vi "Read Attributes.vi"(0 "Linked List in":refnum<class "Linked List.lvclass">, 1 "Linked List ID":string, 3 "Include Private?":bool, 5 "Attribute Names":string[](array[string]), 9 "Flatten Pointer?":bool, 11 "error in (no error)":errorcluster) -> (4 "Linked List out":refnum<class "Linked List.lvclass">, 6 "Attribute Names out":string[](array[string]), 8 "Missing GUIDs out":string[](array[string]), 10 "Attributes":variant[](array[variant]), 12 "Found?":bool[](array[boolean]), 14 "Data IDs":string[](array[string]), 15 "error out":errorcluster)   [LabVIEW 2020, in "Linked Lists.lvlib" / "Linked List.lvclass"]
uses:
  <vilib>/gpm_packages/@cs/linked-list/Source/Linked List/Linked List/Linked List.lvclass
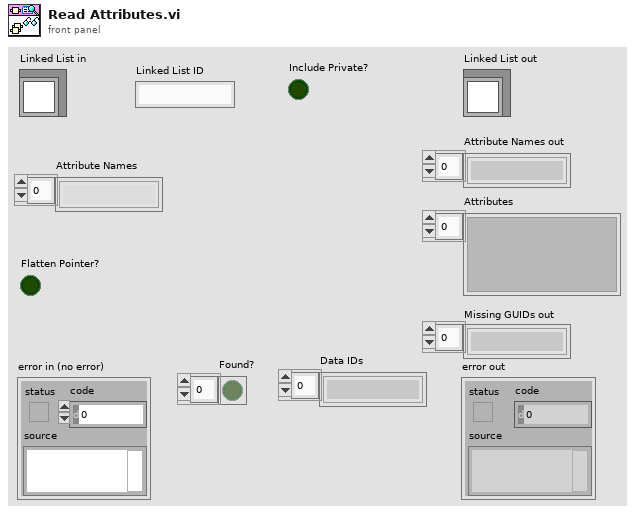
[diagram p1: front panel]
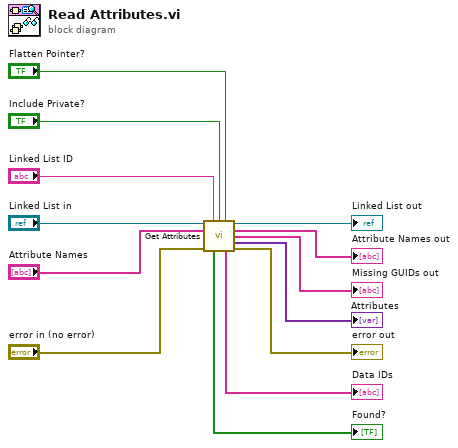
[diagram p0: block diagram]
diagram:
  n1 = call <vilib>:"Get Attributes.vi"("Linked List in"="Linked List in", "Unique ID"="Linked List ID", "Include Private?"="Include Private?", "Flatten Pointer?"="Flatten Pointer?", "Attribute Names"="Attribute Names", "error in (no error)"="error in (no error)") -> ("Linked List out"=→"Linked List out":refnum<class "Linked List.lvclass">, "Attribute Names out"=→"Attribute Names out":string[], "Missing GUIDs out"=→"Missing GUIDs out":string[], "Attributes"=→"Attributes":variant[], "Found?"=→"Found?":bool[], "Data IDs"=→"Data IDs":string[], "error out"=→"error out":errorcluster)  [unwired: 3 in]
